vi "Set Plot Visibility (WDTWFGraph).vi"(8 "error in (no error)":errorcluster, 10 "Plot.Visible?":bool[](array[boolean]), 11 "WFGraph (WDT) in":refnum<vi>) -> (0 "error out":errorcluster)   [LabVIEW 2019, in "Instrument.Lockin.lvlib" / "Instrument UI.Lockin.lvclass"]
uses:
  Instrument UI.Lockin.lvclass
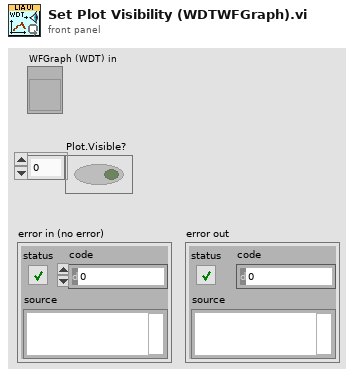
[diagram p1: front panel]
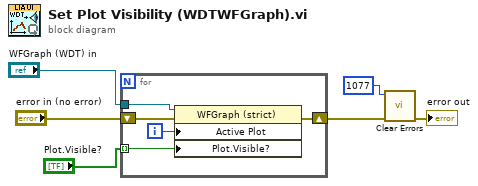
[diagram p0: block diagram]
diagram:
  n1 = for {
    tunnel: "WFGraph (WDT) in" -> [w11]
    shift-right: [w9] -> w3
    shift-left: "error in (no error)" -> [w10]
    tunnel: "Plot.Visible?" -> [w8] mode=indexing
    i -> [w7]
    n2 = property on="Property Node" class="WFGraph (strict)"(reference=w11, error in=w10, "Active Plot"=w7, "Plot.Visible?"=w8) -> (error out=w9:errorcluster)  [unwired: 1 out]
  }
  n3 = call <vilib>:"Clear Errors.vi"("error in (no error)"=w3, "specific error code to clear (0: all)"=1077) -> ("error out"=→"error out":errorcluster)  [unwired: 4 in, 1 out]
